vi "Route.vi"(8 "error in (no error)":errorcluster, 9 "Connect":bool, 10 "Route":string, 11 "reference in":refnum<class "Switch_Manager.lvclass">) -> (0 "error out":errorcluster, 3 "reference in":refnum<class "Switch_Manager.lvclass">)   [LabVIEW 2022 SP3, in "Switch_Manager.lvlib" / "Switch_Manager.lvclass"]
uses:
  Switch_Manager.lvclass
  Components/SwitchBase.lvlibp/SwitchBase.lvclass
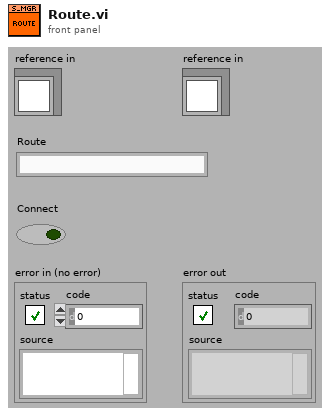
[diagram p1: front panel]
types:
  T1 = typedef "Switch_Manager.lvlib/Switch_Manager.lvclass/ObjectAttributes.ctl" = cluster{"Config":T2, "State":bool[], "Switches":refnum<class "SwitchBase.lvclass">[], "SwitchName":string[], "SwitchMap":T3[], "UpdateEvent":refnum<user-event>, "ParentEvent":refnum<user-event>, "Tree":bool[]}
  T2 = typedef "Switch_Manager.lvlib/Switch_Manager.lvclass/Config.ctl" = cluster{"default":string}
  T3 = typedef "Switch_Manager.lvlib/Switch_Manager.lvclass/SwitchMap.ctl" = cluster{"Name":string, "Description":string, "Group":string, "IsGroup":bool, "Switches":string[]}
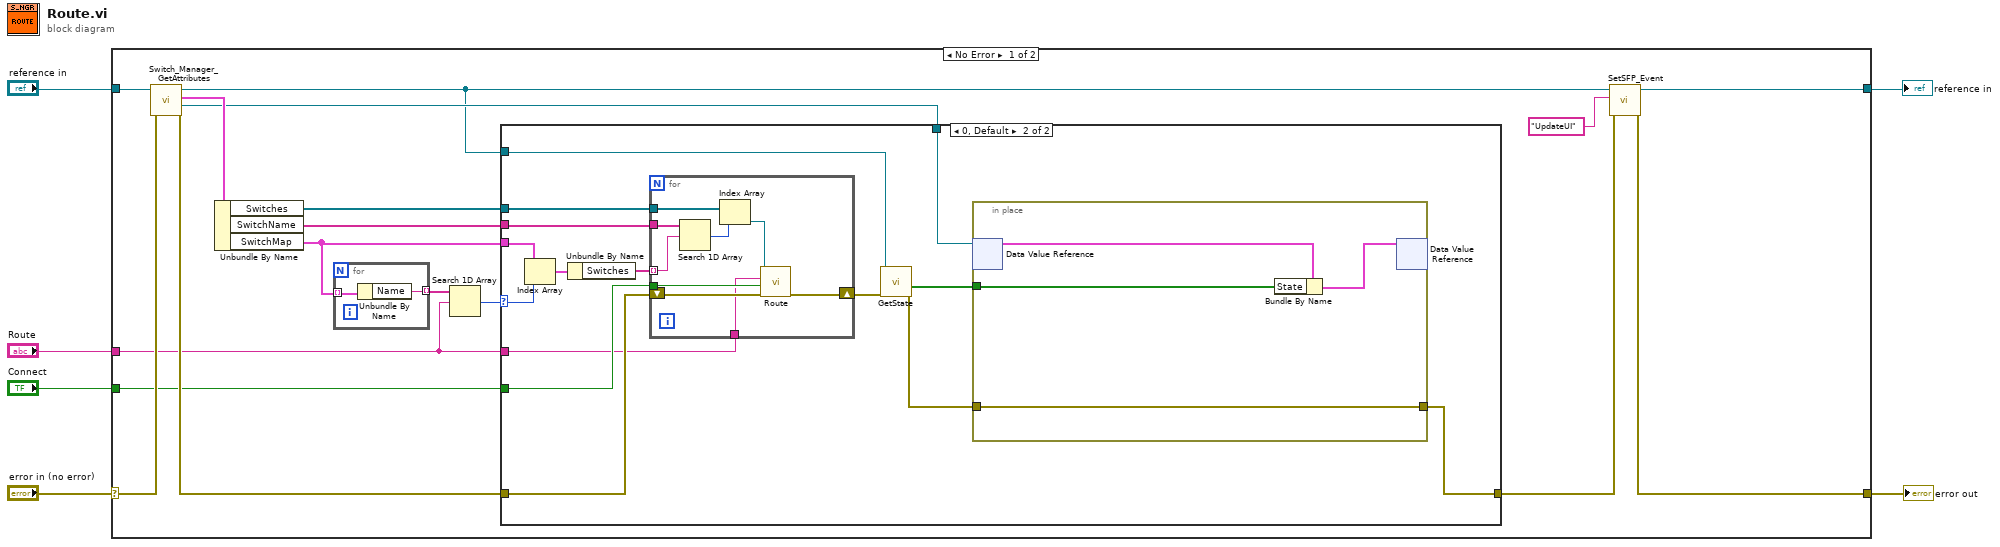
[diagram p0: block diagram]
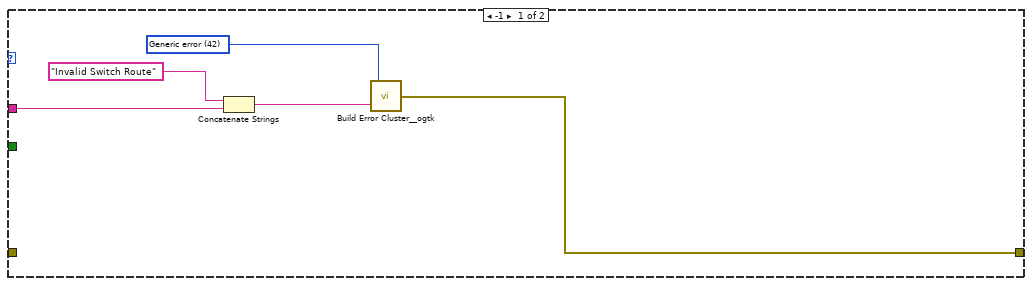
[diagram p2: hidden frame]
diagram:
  n1 = case shown="No Error" "error in (no error)" {
    selector: "error in (no error)" -> [w23 w60]
    tunnel: [w12 w60] -> w5
    tunnel: [w8 w59] -> w3
    tunnel: "reference in" -> [w21 w59]
    tunnel: "Route" -> [w14 _]
    tunnel: "Connect" -> [w15 _]
    frame No Error {
      n2 = call "Switch_Manager_GetAttributes.vi"("error in (no error)"=w23, "reference in"=w21) -> ("error out"=w20:errorcluster, "DataRef"=w11:refnum<data-value>, "Data"=w22:T1, "reference out"=w7:refnum<class "Switch_Manager.lvclass">)  [unwired: 6 in]
      n3 = Unbundle By Name(w22) -> ("Switches"=w9:refnum<class "SwitchBase.lvclass">[], "SwitchName"=w10:string[], "SwitchMap"=w16:T3[])
      n4 = for {
        tunnel: w16 -> [w25] mode=indexing
        tunnel: [w24] -> w18 mode=indexing
        n5 = Unbundle By Name(w25) -> ("Name"=w24:string)
      }
      n6 = Search 1D Array(1D array=w18, element=w14) -> (index of element=w17:i32)  [unwired: 1 in]
      n7 = case shown="0, Default" w17 {
        selector: w17 -> [_ w43]
        tunnel: w20 -> [_ w41]
        tunnel: [w26 w35] -> w13
        tunnel: w14 -> [w29 w36]
        tunnel: w16 -> [_ w45]
        tunnel: w15 -> [_ w40]
        tunnel: w11 -> [_ w42]
        tunnel: w10 -> [_ w38]
        tunnel: w9 -> [_ w37]
        tunnel: w7 -> [_ w33]
        frame -1 {
          w30 = 42 items=["No error", "Argument error", "Memory is full", "Out of zone", "End of file", "File already open", "Generic file I/O error", "File not found", "File permission error", "Disk is full", "Duplicate path", "Too many files open", "System feature not enabled", "Resource file not found", "Cannot add resource", "Resource not found", "Image not found", "Image memory error", "Pen does not exist", "Config type invalid", "Config token not found", "Config parse error", "Config memory error", "Bad external code format", "Bad external code offset", "External code not present", "Null window", "Destroy window error", "Null menu", "Print aborted", "Bad print record", "Print driver error", "Windows error during printing", "Memory error during printing", "Print dialog error", "Generic print error", "Invalid device refnum", "Device not found", "Device parameter error", "Device unit error", "Cannot open device", "Device call aborted", "Generic error", "Cancelled by user", "Object ID too low", "Object ID too high", "Object not in heap", "Unknown heap", "Unknown object (invalid DefProc)", "Unknown object (DefProc not in table)", "Message out of range", "Invalid (null) method", "Unknown message", "Manager call not supported", "Bad address", "Network operation in progress", "Network operation timed out", "Connection is busy", "Network attribute not supported", "Network error", "Address in use", "System out of memory", "Connection aborted", "Connection refused", "Not connected", "Already connected", "Connection closed", "Initialization error (interapplication manager)", "Bad occurrence", "Wait on unbound occurrence handler", "Occurrence queue overflow", "Datalog type conflict", "Unused", "Unrecognized type (interapplication manager)", "Memory corrupt", "Failed to make temporary DLL", "Old CIN version", "Drag socket not found", "Failed to load drop-object", "Failed to register OLE object", "Failed to release OLE object", "Format specifier type mismatch", "Unknown format specifier", "Too few format specifiers", "Too many format specifiers", "Scan failed", "Newer CIN version", "Error converting to variant", "Runtime menu error", "Password tampered", "Variant attribute not found", "Incompatible variant data type", "Event data is not available", "Event Store is not present", "Occurrence is not found", "Event Queue is not created", "Event info is not available", "Refnum passed is NULL", "Error retrieving Class GUID", "Error retrieving CoClass GUID", "Error retrieving TypeLib GUID.", "Bad built application magic bytes.", "Specific driver is different from the specific driver associated with the Logical Name.", "There is no session opened to the class driver.", "Max Error", "MAX - Error with config objects", "MAX - Error loading configuration", "MAX - Group not supported"]
          n8 = Concatenate Strings("Invalid Switch Route" ("string"), w29) -> (w27:string)
          n9 = call <userlib>:"Build Error Cluster__ogtk.vi"("String to Prepend to source (\"\")"=w27, "code"=w30) -> ("error out"=w26:errorcluster)
        }
        frame 0, Default {
          n10 = Index Array(array=w45, index=w43) -> (element=w44:T3)
          n11 = Unbundle By Name(w44) -> ("Switches"=w39:string[])
          n12 = for {
            shift-right: [w52] -> w34
            shift-left: w41 -> [w54]
            tunnel: w40 -> [w53]
            tunnel: w39 -> [w51] mode=indexing
            tunnel: w38 -> [w50]
            tunnel: w37 -> [w49]
            tunnel: w36 -> [w47]
            n13 = Search 1D Array(1D array=w50, element=w51) -> (index of element=w48:i32)  [unwired: 1 in]
            n14 = Index Array(array=w49, index=w48) -> (element=w46:refnum<class "SwitchBase.lvclass">)
            n15 = call-dynamic "Route.vi"("error in (no error)"=w54, "Connect"=w53, "channel 1"=w47, "reference in"=w46) -> ("error out"=w52:errorcluster)  [unwired: 6 in, 1 out]
          }
          n16 = call-dynamic "GetState.vi"("error in (no error)"=w34, "reference in"=w33) -> ("error out"=w32:errorcluster, "States"=w31:bool[])  [unwired: 6 in, 2 out]
          n17 = in-place {
            in-place-border: [w56] -> w35
            in-place-border: w32 -> [w56]
            in-place-border: w31 -> [w55]
            n18 = in-place-dvr #1(w42) -> (w58:T1)  [unwired: 1 out]
            n19 = Bundle By Name(cluster=w58, "State"=w55) -> (w57:T1)
            n20 = in-place-dvr #1(w57) -> ()  [unwired: 2 out]
          }
        }
      }
      n21 = call-dynamic "SetSFP_Event.vi"("error in (no error)"=w13, "msg"="UpdateUI", "reference in"=w7) -> ("error out"=w12:errorcluster, "reference out"=w8:refnum<class "Switch_Manager.lvclass">)  [unwired: 7 in]
    }
    frame Error {
    }
  }
  "error out" <- w5
  "reference in" <- w3
